vi "PulseGenEPTx_Spark.vi"(0 "Spark_Config":T3, 4 "Spark_Sequences":T1(array[cluster]), 7 "EPTxSupervisor":T2) -> (20 "CmdOut1":bool, 21 "CmdOut2":bool, 22 "CmdOut3":bool, 23 "CmdOut4":bool, 24 "CmdOut5":bool, 25 "CmdOut6":bool, 26 "CmdOut7":bool, 27 "CmdOut8":bool)   [LabVIEW 2015]
doc: "This VI is used to generate a sequence with at least one pulse with variable dwell for up to eight spark channels. In addition to the main pulse, the command sequence block enables three additional time-based pulses intended for spark re-strike. The Spark_Config cluster sets the channel enable, firing window, main timing (end-angle), and main dwell for each channel separately. The indivudual channel command sequences are configured in the Spark_Sequences array of clusters. This VI is supervised by the EPTxSupervisor cluster."
uses:
  <vilib>/Powertrain Controls/Device Drivers/Engine Position Tracking/EPTx/RevA/FPGA/Controls/EPTxSupervisor.ctl
  <vilib>/Powertrain Controls/Device Drivers/Engine Position Tracking/EPTx/RevA/FPGA/Controls/EPTxAOSAControl.ctl
  <vilib>/Powertrain Controls/Device Drivers/Engine Position Tracking/EPTx/RevA/FPGA/Controls/EPTxAAPControl.ctl
  <vilib>/Powertrain Controls/Device Drivers/Engine Position Tracking/EPTx/RevA/FPGA/Extras/Command Sequence - 16e.vi
  <vilib>/Powertrain Controls/Device Drivers/Engine Position Tracking/EPTx/RevA/FPGA/Extras/Angle One Shot With Advance - 8x - Multi.vi
  <vilib>/Powertrain Controls/Device Drivers/Engine Position Tracking/EPTx/RevA/FPGA/EPTx - RevA - FPGA.lvlib
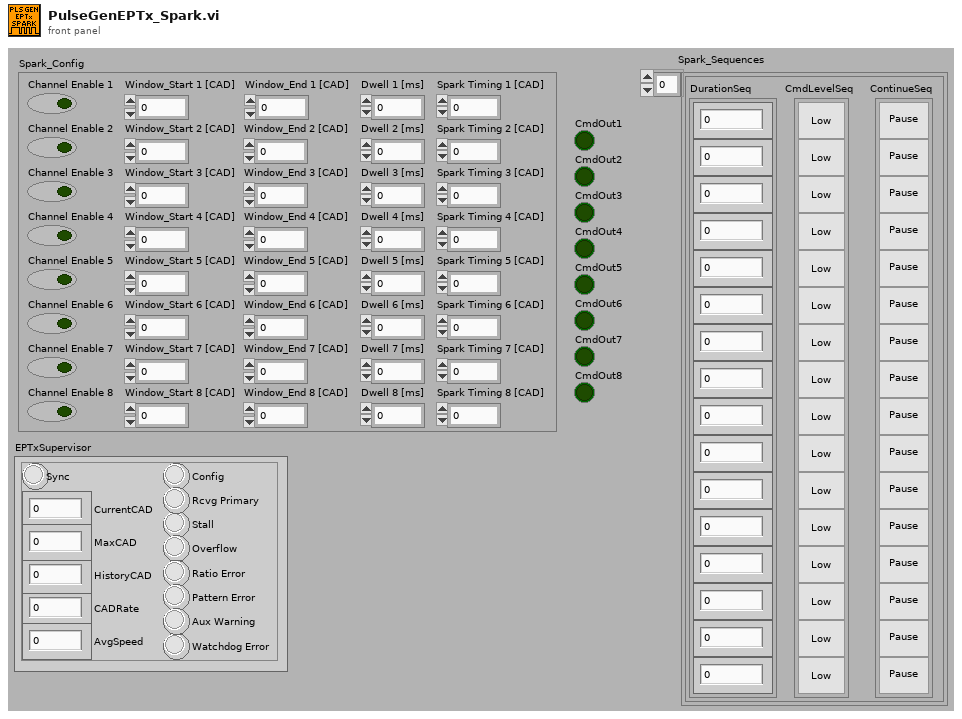
[diagram p1: front panel]
types:
  T1 = cluster{"DurationSeq":u32[], "CmdLevelSeq":bool[], "ContinueSeq":bool[]}[]
  T2 = typedef "EPTx - RevA - FPGA.lvlib/EPTxSupervisor.ctl" = cluster{"Sync":bool, "CurrentCAD":fxp<+,18,11>, "MaxCAD":fxp<+,11,11>, "HistoryCAD":fxp<+,11,11>, "CADRate":fxp<+,22,8>, "AvgSpeed":fxp<+,17,15>, "Config":bool, "Rcvg Primary":bool, "Stall":bool, "Overflow":bool, "Ratio Error":bool, "Pattern Error":bool, "Aux Warning":bool, "Watchdog Error":bool}
  T3 = cluster{"Channel Enable 1":bool, "Window_Start 1 [CAD]":fxp<+,18,11>, "Window_End 1 [CAD]":fxp<+,18,11>, "Dwell 1 [ms]":fxp<+/-,22,9>, "Spark Timing 1 [CAD]":fxp<+,18,11>, "Channel Enable 2":bool, "Window_Start 2 [CAD]":fxp<+,18,11>, "Window_End 2 [CAD]":fxp<+,18,11>, "Dwell 2 [ms]":fxp<+/-,22,9>, "Spark Timing 2 [CAD]":fxp<+,18,11>, "Channel Enable 3":bool, "Window_Start 3 [CAD]":fxp<+,18,11>, "Window_End 3 [CAD]":fxp<+,18,11>, "Dwell 3 [ms]":fxp<+/-,22,9>, "Spark Timing 3 [CAD]":fxp<+,18,11>, "Channel Enable 4":bool, "Window_Start 4 [CAD]":fxp<+,18,11>, "Window_End 4 [CAD]":fxp<+,18,11>, "Dwell 4 [ms]":fxp<+/-,22,9>, "Spark Timing 4 [CAD]":fxp<+,18,11>, "Channel Enable 5":bool, "Window_Start 5 [CAD]":fxp<+,18,11>, "Window_End 5 [CAD]":fxp<+,18,11>, "Dwell 5 [ms]":fxp<+/-,22,9>, "Spark Timing 5 [CAD]":fxp<+,18,11>, "Channel Enable 6":bool, "Window_Start 6 [CAD]":fxp<+,18,11>, "Window_End 6 [CAD]":fxp<+,18,11>, "Dwell 6 [ms]":fxp<+/-,22,9>, "Spark Timing 6 [CAD]":fxp<+,18,11>, "Channel Enable 7":bool, "Window_Start 7 [CAD]":fxp<+,18,11>, "Window_End 7 [CAD]":fxp<+,18,11>, "Dwell 7 [ms]":fxp<+/-,22,9>, "Spark Timing 7 [CAD]":fxp<+,18,11>, "Channel Enable 8":bool, "Window_Start 8 [CAD]":fxp<+,18,11>, "Window_End 8 [CAD]":fxp<+,18,11>, "Dwell 8 [ms]":fxp<+/-,22,9>, "Spark Timing 8 [CAD]":fxp<+,18,11>}
  T4 = typedef "EPTx - RevA - FPGA.lvlib/EPTxAAPControl.ctl" = cluster{"Enable":bool, "RisingCAD":fxp<+,18,11>, "FallingCAD":fxp<+,18,11>}
  T5 = typedef "EPTx - RevA - FPGA.lvlib/EPTxAOSAControl.ctl" = cluster{"Enable":bool, "OneShotCAD":fxp<+,18,11>, "OneShotAdvance":fxp<+/-,22,9>}
  T6 = cluster{"DurationSeq":u32[], "CmdLevelSeq":bool[], "ContinueSeq":bool[]}
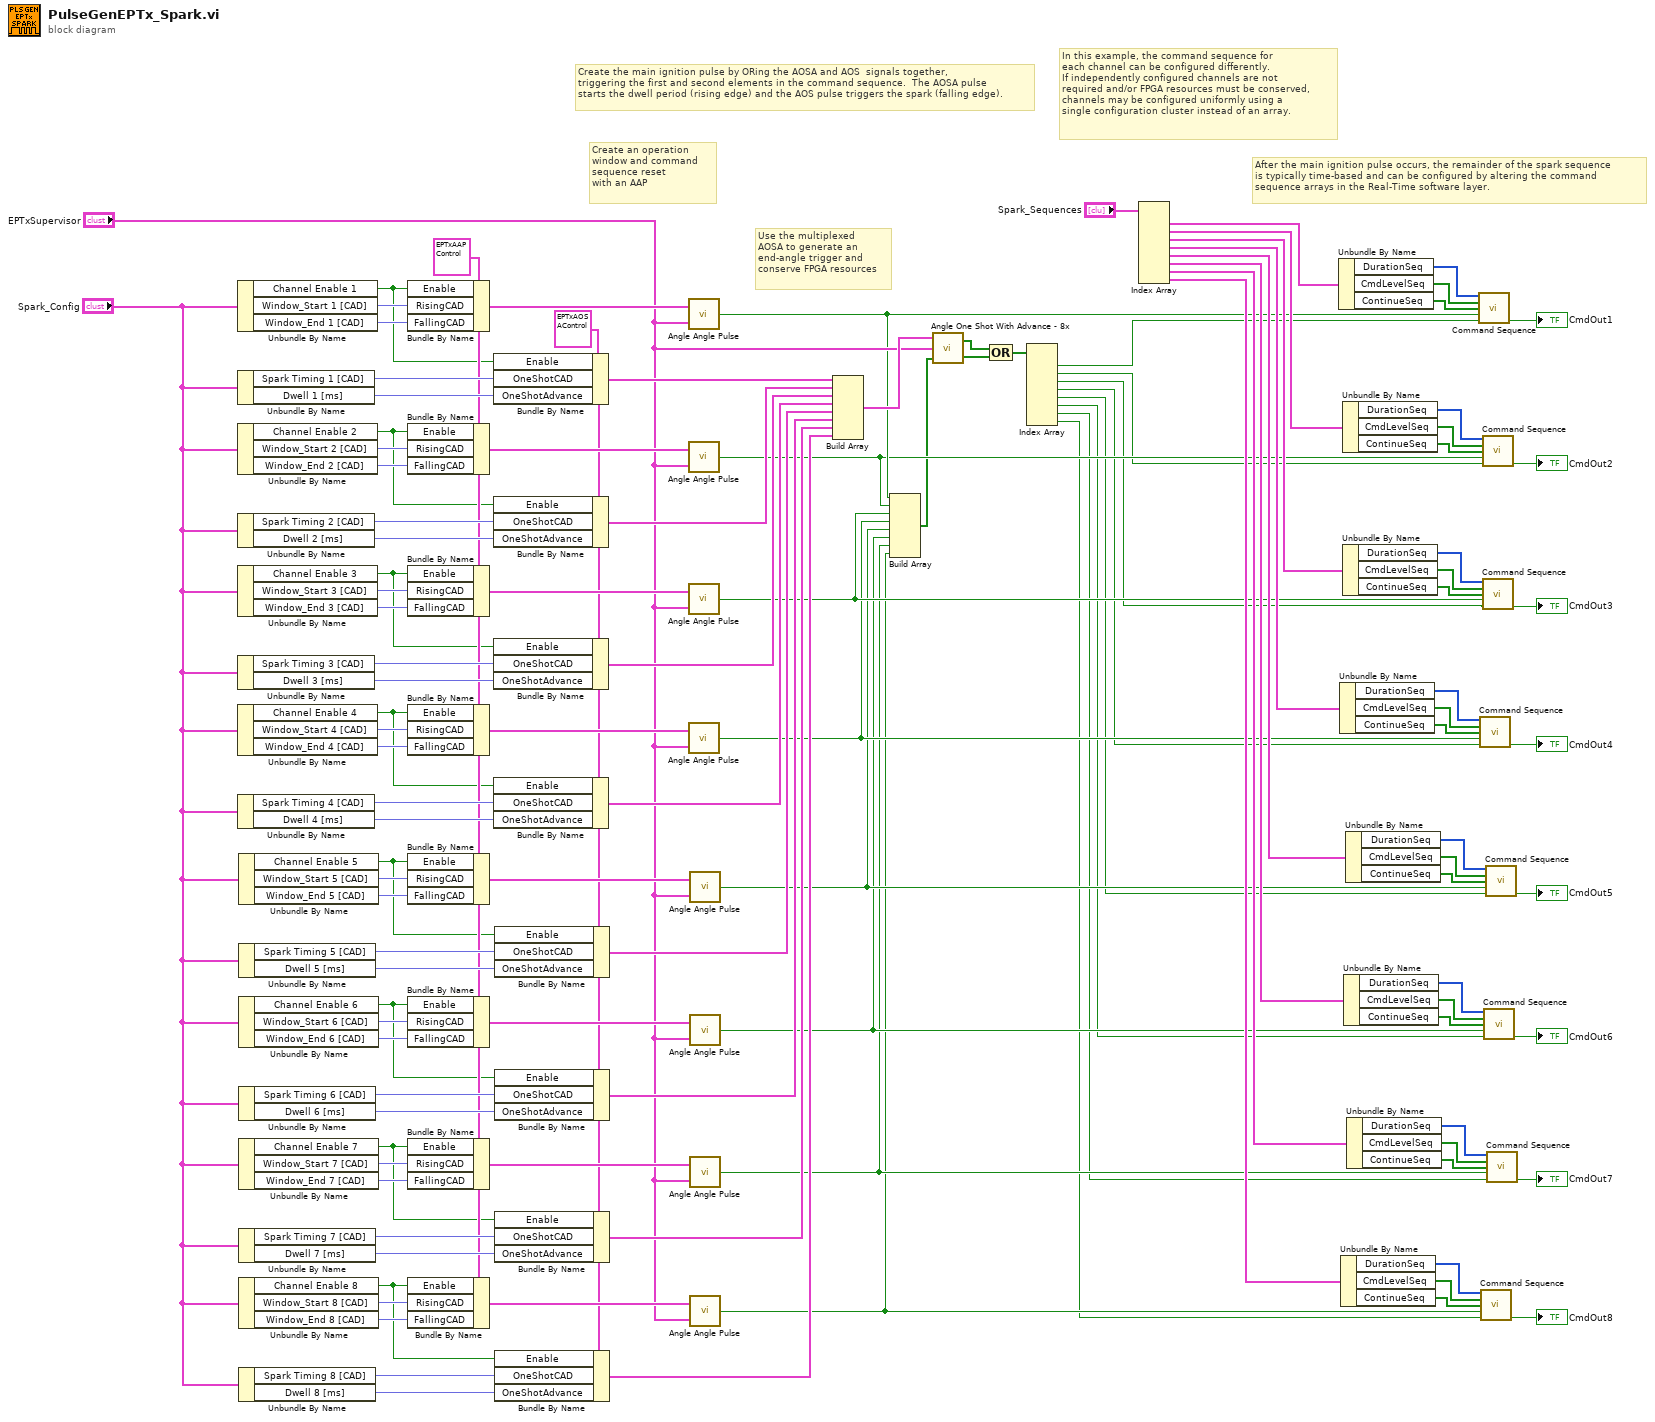
[diagram p0: block diagram]
diagram:
  w49 = T4 {"Enable"=FALSE, "RisingCAD"=0.0, "FallingCAD"=0.0} ("AAPControl")
  w48 = T5 {"Enable"=FALSE, "OneShotCAD"=0.0, "OneShotAdvance"=0.0} ("AOSAControl")
  # "Use the multiplexed\nAOSA to generate an \nend-angle trigger and\nconserve FPGA resources"
  # "In this example, the command sequence for\neach channel can be configured differently.  \nIf independently configured channels are not \nrequired and/or FPGA resources must be conserved,\nchannels may be configured uniformly using a\nsingle configuration cluster instead of an array."
  # "After the main ignition pulse occurs, the remainder of the spark sequence \nis typically time-based and can be configured by altering the command \nsequence arrays in the Real-Time software layer."
  # "Create the main ignition pulse by ORing the AOSA and AOS  signals together, \ntriggering the first and second elements in the command sequence.  The AOSA pulse \nstarts the dwell period (rising edge) and the AOS pulse triggers the spark (falling edge)."
  # "Create an operation\nwindow and command\nsequence reset\nwith an AAP"
  n1 = Unbundle By Name("Spark_Config") -> ("Channel Enable 1"=w40:bool, "Window_Start 1 [CAD]"=w121:fxp<+,18,11>, "Window_End 1 [CAD]"=w120:fxp<+,18,11>)
  n2 = Unbundle By Name("Spark_Config") -> ("Spark Timing 1 [CAD]"=w119:fxp<+,18,11>, "Dwell 1 [ms]"=w118:fxp<+/-,22,9>)
  n3 = Unbundle By Name("Spark_Config") -> ("Channel Enable 2"=w41:bool, "Window_Start 2 [CAD]"=w114:fxp<+,18,11>, "Window_End 2 [CAD]"=w115:fxp<+,18,11>)
  n4 = Unbundle By Name("Spark_Config") -> ("Spark Timing 2 [CAD]"=w116:fxp<+,18,11>, "Dwell 2 [ms]"=w117:fxp<+/-,22,9>)
  n5 = Unbundle By Name("Spark_Config") -> ("Channel Enable 3"=w42:bool, "Window_Start 3 [CAD]"=w112:fxp<+,18,11>, "Window_End 3 [CAD]"=w111:fxp<+,18,11>)
  n6 = Unbundle By Name("Spark_Config") -> ("Spark Timing 3 [CAD]"=w110:fxp<+,18,11>, "Dwell 3 [ms]"=w109:fxp<+/-,22,9>)
  n7 = Unbundle By Name("Spark_Config") -> ("Channel Enable 4"=w43:bool, "Window_Start 4 [CAD]"=w105:fxp<+,18,11>, "Window_End 4 [CAD]"=w106:fxp<+,18,11>)
  n8 = Unbundle By Name("Spark_Config") -> ("Spark Timing 4 [CAD]"=w107:fxp<+,18,11>, "Dwell 4 [ms]"=w108:fxp<+/-,22,9>)
  n9 = Unbundle By Name("Spark_Config") -> ("Channel Enable 5"=w44:bool, "Window_Start 5 [CAD]"=w85:fxp<+,18,11>, "Window_End 5 [CAD]"=w86:fxp<+,18,11>)
  n10 = Unbundle By Name("Spark_Config") -> ("Spark Timing 5 [CAD]"=w87:fxp<+,18,11>, "Dwell 5 [ms]"=w88:fxp<+/-,22,9>)
  n11 = Unbundle By Name("Spark_Config") -> ("Channel Enable 6"=w45:bool, "Window_Start 6 [CAD]"=w92:fxp<+,18,11>, "Window_End 6 [CAD]"=w91:fxp<+,18,11>)
  n12 = Unbundle By Name("Spark_Config") -> ("Spark Timing 6 [CAD]"=w90:fxp<+,18,11>, "Dwell 6 [ms]"=w89:fxp<+/-,22,9>)
  n13 = Unbundle By Name("Spark_Config") -> ("Channel Enable 7"=w46:bool, "Window_Start 7 [CAD]"=w95:fxp<+,18,11>, "Window_End 7 [CAD]"=w96:fxp<+,18,11>)
  n14 = Unbundle By Name("Spark_Config") -> ("Spark Timing 7 [CAD]"=w97:fxp<+,18,11>, "Dwell 7 [ms]"=w98:fxp<+/-,22,9>)
  n15 = Unbundle By Name("Spark_Config") -> ("Channel Enable 8"=w47:bool, "Window_Start 8 [CAD]"=w102:fxp<+,18,11>, "Window_End 8 [CAD]"=w101:fxp<+,18,11>)
  n16 = Unbundle By Name("Spark_Config") -> ("Spark Timing 8 [CAD]"=w100:fxp<+,18,11>, "Dwell 8 [ms]"=w99:fxp<+/-,22,9>)
  n17 = Bundle By Name(cluster=w49, "Enable"=w40, "RisingCAD"=w121, "FallingCAD"=w120) -> (w122:T4)
  n18 = Bundle By Name(cluster=w49, "Enable"=w41, "RisingCAD"=w114, "FallingCAD"=w115) -> (w50:T4)
  n19 = Bundle By Name(cluster=w49, "Enable"=w42, "RisingCAD"=w112, "FallingCAD"=w111) -> (w113:T4)
  n20 = Bundle By Name(cluster=w49, "Enable"=w43, "RisingCAD"=w105, "FallingCAD"=w106) -> (w104:T4)
  n21 = Bundle By Name(cluster=w49, "Enable"=w44, "RisingCAD"=w85, "FallingCAD"=w86) -> (w84:T4)
  n22 = Bundle By Name(cluster=w49, "Enable"=w45, "RisingCAD"=w92, "FallingCAD"=w91) -> (w93:T4)
  n23 = Bundle By Name(cluster=w49, "Enable"=w46, "RisingCAD"=w95, "FallingCAD"=w96) -> (w94:T4)
  n24 = Bundle By Name(cluster=w49, "Enable"=w47, "RisingCAD"=w102, "FallingCAD"=w101) -> (w103:T4)
  n25 = Bundle By Name(cluster=w48, "Enable"=w40, "OneShotCAD"=w119, "OneShotAdvance"=w118) -> (w30:T5)
  n26 = Bundle By Name(cluster=w48, "Enable"=w41, "OneShotCAD"=w116, "OneShotAdvance"=w117) -> (w29:T5)
  n27 = Bundle By Name(cluster=w48, "Enable"=w42, "OneShotCAD"=w110, "OneShotAdvance"=w109) -> (w28:T5)
  n28 = Bundle By Name(cluster=w48, "Enable"=w43, "OneShotCAD"=w107, "OneShotAdvance"=w108) -> (w27:T5)
  n29 = Bundle By Name(cluster=w48, "Enable"=w44, "OneShotCAD"=w87, "OneShotAdvance"=w88) -> (w26:T5)
  n30 = Bundle By Name(cluster=w48, "Enable"=w45, "OneShotCAD"=w90, "OneShotAdvance"=w89) -> (w25:T5)
  n31 = Bundle By Name(cluster=w48, "Enable"=w46, "OneShotCAD"=w97, "OneShotAdvance"=w98) -> (w24:T5)
  n32 = Bundle By Name(cluster=w48, "Enable"=w47, "OneShotCAD"=w100, "OneShotAdvance"=w99) -> (w23:T5)
  n33 = call <vilib>:"Angle Angle Pulse.vi"("EPTxSupervisor"="EPTxSupervisor", "AAPControl"=w122) -> ("AAP"=w20:bool)
  n34 = call <vilib>:"Angle Angle Pulse.vi"("EPTxSupervisor"="EPTxSupervisor", "AAPControl"=w50) -> ("AAP"=w19:bool)
  n35 = call <vilib>:"Angle Angle Pulse.vi"("EPTxSupervisor"="EPTxSupervisor", "AAPControl"=w113) -> ("AAP"=w18:bool)
  n36 = call <vilib>:"Angle Angle Pulse.vi"("EPTxSupervisor"="EPTxSupervisor", "AAPControl"=w104) -> ("AAP"=w17:bool)
  n37 = call <vilib>:"Angle Angle Pulse.vi"("EPTxSupervisor"="EPTxSupervisor", "AAPControl"=w84) -> ("AAP"=w16:bool)
  n38 = call <vilib>:"Angle Angle Pulse.vi"("EPTxSupervisor"="EPTxSupervisor", "AAPControl"=w93) -> ("AAP"=w15:bool)
  n39 = call <vilib>:"Angle Angle Pulse.vi"("EPTxSupervisor"="EPTxSupervisor", "AAPControl"=w94) -> ("AAP"=w14:bool)
  n40 = call <vilib>:"Angle Angle Pulse.vi"("EPTxSupervisor"="EPTxSupervisor", "AAPControl"=w103) -> ("AAP"=w13:bool)
  n41 = Build Array(w30, w29, w28, w27, w26, w25, w24, w23) -> (w22:T5[])
  n42 = Build Array(w20, w19, w18, w17, w16, w15, w14, w13) -> (w1:bool[])
  n43 = call-poly <vilib>:"Angle One Shot With Advance - 8x.vi"("OpWindow Array"=w1, "EPTxSupervisor"="EPTxSupervisor", "AOSAControl"=w22) -> ("AOS"=w11:bool[], "AOSAdv"=w12:bool[])
  n44 = Compound Arithmetic op=OR(w12, w11) -> (w7:bool[])
  n45 = Index Array(array=w7) -> (element #1=w10:bool, element #2=w8:bool, element #3=w9:bool, element #4=w6:bool, element #5=w5:bool, element #6=w4:bool, element #7=w3:bool, element #8=w2:bool)  [unwired: 8 in]
  n46 = Index Array(array="Spark_Sequences") -> (element #1=w38:T6, element #2=w37:T6, element #3=w36:T6, element #4=w35:T6, element #5=w33:T6, element #6=w34:T6, element #7=w32:T6, element #8=w31:T6)  [unwired: 8 in]
  n47 = Unbundle By Name(w38) -> ("DurationSeq"=w82:u32[], "CmdLevelSeq"=w81:bool[], "ContinueSeq"=w80:bool[])
  n48 = Unbundle By Name(w35) -> ("DurationSeq"=w72:u32[], "CmdLevelSeq"=w73:bool[], "ContinueSeq"=w74:bool[])
  n49 = Unbundle By Name(w31) -> ("DurationSeq"=w60:u32[], "CmdLevelSeq"=w61:bool[], "ContinueSeq"=w62:bool[])
  n50 = Unbundle By Name(w37) -> ("DurationSeq"=w78:u32[], "CmdLevelSeq"=w79:bool[], "ContinueSeq"=w51:bool[])
  n51 = Unbundle By Name(w36) -> ("DurationSeq"=w77:u32[], "CmdLevelSeq"=w76:bool[], "ContinueSeq"=w75:bool[])
  n52 = Unbundle By Name(w34) -> ("DurationSeq"=w66:u32[], "CmdLevelSeq"=w67:bool[], "ContinueSeq"=w68:bool[])
  n53 = Unbundle By Name(w33) -> ("DurationSeq"=w71:u32[], "CmdLevelSeq"=w70:bool[], "ContinueSeq"=w69:bool[])
  n54 = Unbundle By Name(w32) -> ("DurationSeq"=w65:u32[], "CmdLevelSeq"=w64:bool[], "ContinueSeq"=w63:bool[])
  n55 = call-poly <vilib>:"Command Sequence.vi"("DurationSeq"=w82, "CmdLevelSeq"=w81, "ContinueSeq"=w80, "SeqReset"=w20, "GlobalTrigger"=w10) -> ("Cmd"=→"CmdOut1":bool)  [unwired: 7 in, 3 out]
  n56 = call-poly <vilib>:"Command Sequence.vi"("DurationSeq"=w72, "CmdLevelSeq"=w73, "ContinueSeq"=w74, "SeqReset"=w17, "GlobalTrigger"=w6) -> ("Cmd"=→"CmdOut4":bool)  [unwired: 7 in, 3 out]
  n57 = call-poly <vilib>:"Command Sequence.vi"("DurationSeq"=w60, "CmdLevelSeq"=w61, "ContinueSeq"=w62, "SeqReset"=w13, "GlobalTrigger"=w2) -> ("Cmd"=→"CmdOut8":bool)  [unwired: 7 in, 3 out]
  n58 = call-poly <vilib>:"Command Sequence.vi"("DurationSeq"=w78, "CmdLevelSeq"=w79, "ContinueSeq"=w51, "SeqReset"=w19, "GlobalTrigger"=w8) -> ("Cmd"=→"CmdOut2":bool)  [unwired: 7 in, 3 out]
  n59 = call-poly <vilib>:"Command Sequence.vi"("DurationSeq"=w77, "CmdLevelSeq"=w76, "ContinueSeq"=w75, "SeqReset"=w18, "GlobalTrigger"=w9) -> ("Cmd"=→"CmdOut3":bool)  [unwired: 7 in, 3 out]
  n60 = call-poly <vilib>:"Command Sequence.vi"("DurationSeq"=w66, "CmdLevelSeq"=w67, "ContinueSeq"=w68, "SeqReset"=w15, "GlobalTrigger"=w4) -> ("Cmd"=→"CmdOut6":bool)  [unwired: 7 in, 3 out]
  n61 = call-poly <vilib>:"Command Sequence.vi"("DurationSeq"=w71, "CmdLevelSeq"=w70, "ContinueSeq"=w69, "SeqReset"=w16, "GlobalTrigger"=w5) -> ("Cmd"=→"CmdOut5":bool)  [unwired: 7 in, 3 out]
  n62 = call-poly <vilib>:"Command Sequence.vi"("DurationSeq"=w65, "CmdLevelSeq"=w64, "ContinueSeq"=w63, "SeqReset"=w14, "GlobalTrigger"=w3) -> ("Cmd"=→"CmdOut7":bool)  [unwired: 7 in, 3 out]
